vi "Counter - Count Edges.vi"() -> ()   [LabVIEW 2017]
doc: "本范例演示连续读回所有经计数器输入计算到的数字边沿的方法。\n\n关于将信号连接至DAQ设备的方法，可参考设备文档。"
uses:
  <vilib>/Utility/error.llb/DialogType.ctl
  <vilib>/DAQmx/read.llb/DAQmx Read (Counter U32 1Chan 1Samp).vi
  <vilib>/DAQmx/create/channels.llb/DAQmx Create Channel (CI-Count Edges).vi
  <vilib>/DAQmx/miscellaneous.llb/DAQmx Fill In Error Info.vi
  <resource>/objmgr/daqmx.rc
panel:
  in  "有效边沿":i32(ring)=10171 items=["上升"=10280, "下降"=10171]
  out "计数":u32
  in  "输入接线端":tag="PFI8"
  in  "计数器":tag="Dev1/ctr0"
  in  "触发类型":T1(tab)
  in  "边沿":i32(ring)=10280 items=["上升"=10280, "下降"=10171]
  in  "数字触发源":tag
  in  "暂停条件":i32(ring)=10192 items=["高"=10192, "低"=10214]
  in  "暂停触发源":tag
  in  "计数重置接线端":tag
  in  "边沿":i32(ring)=10280 items=["上升"=10280, "下降"=10171]
  in  "停止":bool
  in  "循环时间(ms)":u32=10
  # "采集数据"
  # "通道设置"
  # "定时\n设置"
  # "触发设置"
  # "如需配置并使用触发/计数重置，必须先在上面选择相应的选项卡。  有些硬件不支持上述选项－更多信息见设备的相应文档。"
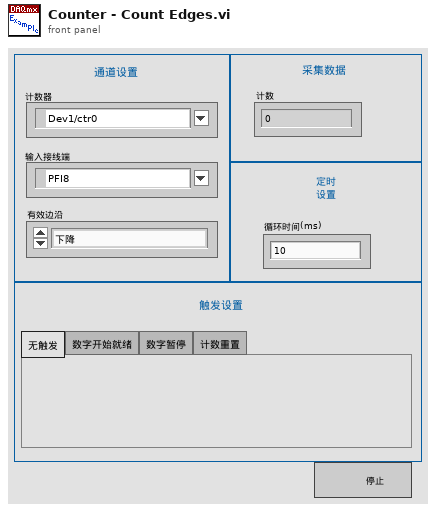
[diagram p1: front panel]
types:
  T1 = enum32{"No Trigger", "Digital Arm Start", "Digital Pause", "Count Reset"}
  T2 = typedef "DialogType.ctl" = u16
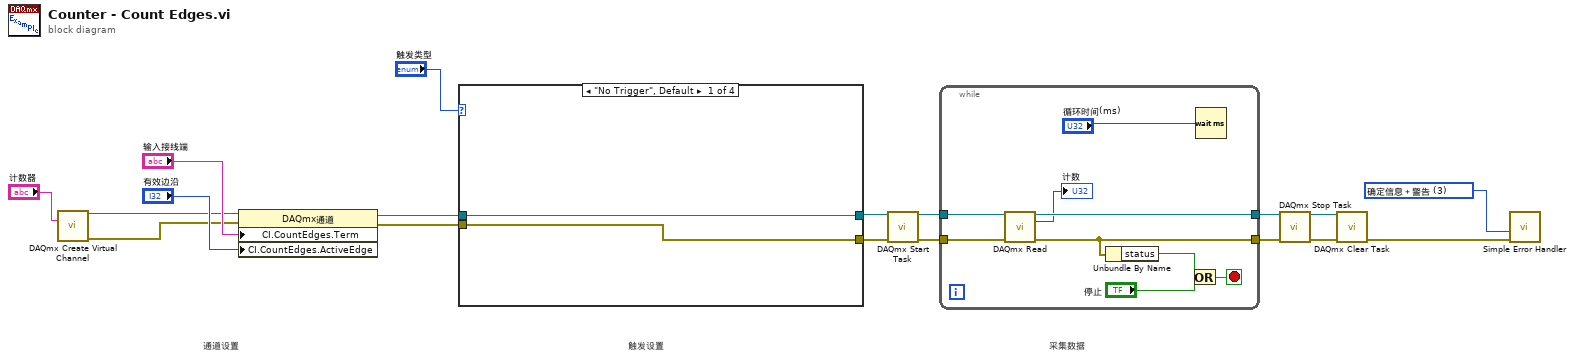
[diagram p0: block diagram]
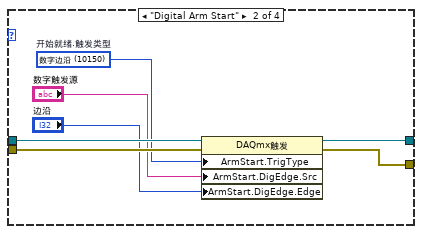
[diagram p2: hidden frame]
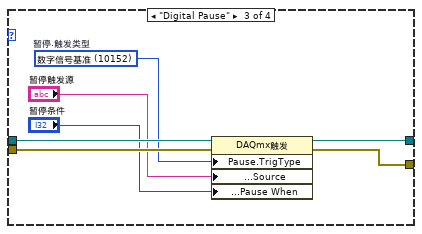
[diagram p3: hidden frame]
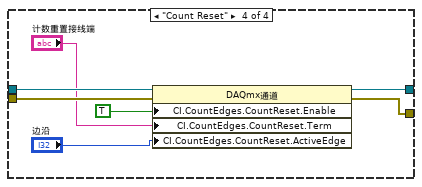
[diagram p4: hidden frame]
diagram:
  w1 = T2 3 items=["无对话框", "确定信息", "继续或停止信息", "确定信息＋警告", "继续/停止＋警告"] ("对话框类型（确定信息：1）")
  # "采集数据"
  # "触发设置"
  # "通道设置"
  n1 = call-poly <vilib>:"DAQmx Create Virtual Channel.vi"("counter"="计数器") -> ("task out"=w9:refnum<k21>, "error out"=w8:errorcluster)  [unwired: 13 in]
  n2 = property class="DAQmx通道"(reference=w9, error in=w8, "CI.CountEdges.Term"="输入接线端", "CI.CountEdges.ActiveEdge"="有效边沿") -> (reference out=w6:refnum<k21>, error out=w7:errorcluster)
  n3 = case shown="\"No Trigger\", Default" "触发类型" {
    tunnel: w6 -> [w20 w27 w34 w41]
    tunnel: w7 -> [w19 w24 w31 w38]
    tunnel: [w20 w26 w33 w40] -> w16
    tunnel: [w19 w25 w32 w39] -> w15
    frame "No Trigger", Default {
    }
    frame "Digital Arm Start" {
      w21 = 10150 items=["数字边沿"=10150, "无"=10230]  # 开始就绪.触发类型
      n4 = property class="DAQmx触发"(reference=w27, error in=w24, "ArmStart.TrigType"=w21, "ArmStart.DigEdge.Src"="数字触发源", "ArmStart.DigEdge.Edge"="边沿") -> (reference out=w26:refnum<k21>, error out=w25:errorcluster)
    }
    frame "Digital Pause" {
      w30 = 10152 items=["模拟信号基准"=10101, "模拟窗"=10103, "数字信号基准"=10152, "数字模式"=10398, "无"=10230]  # 暂停.触发类型
      n5 = property class="DAQmx触发"(reference=w34, error in=w31, "Pause.TrigType"=w30, "More:Pause:Digital Level:Source"="暂停触发源", "More:Pause:Digital Level:Pause When"="暂停条件") -> (reference out=w33:refnum<k21>, error out=w32:errorcluster)
    }
    frame "Count Reset" {
      n6 = property class="DAQmx通道"(reference=w41, error in=w38, "CI.CountEdges.CountReset.Enable"=TRUE ("计数器输入.边沿计数.计数重置.启用"), "CI.CountEdges.CountReset.Term"="计数重置接线端", "CI.CountEdges.CountReset.ActiveEdge"="边沿") -> (reference out=w40:refnum<k21>, error out=w39:errorcluster)
    }
  }
  n7 = call <vilib>:"DAQmx Start Task.vi"("task/channels in"=w16, "error in"=w15) -> ("task out"=w14:refnum<k21>, "error out"=w13:errorcluster)  [unwired: 12 in]
  n8 = while {
    tunnel: w14 -> [w50]
    tunnel: w13 -> [w49]
    tunnel: [w46] -> w4
    tunnel: [w47] -> w5
    stop <- w48 stop-if-true
    n9 = call-poly <vilib>:"DAQmx Read.vi"("task/channels in"=w50, "error in"=w49) -> ("task out"=w47:refnum<k21>, "data"=→"计数":u32, "error out"=w46:errorcluster)  [unwired: 11 in]
    n10 = Unbundle By Name(w46) -> ("status"=w45:bool)
    n11 = Or(x=w45, y="停止") -> (x .or. y?=w48:bool)
    n12 = Wait (ms)(milliseconds to wait="循环时间(ms)") -> ()  [unwired: 1 out]
  }
  n13 = call <vilib>:"DAQmx Stop Task.vi"("task/channels in"=w5, "error in"=w4) -> ("task out"=w2:refnum<k21>, "error out"=w3:errorcluster)  [unwired: 12 in]
  n14 = call <vilib>:"DAQmx Clear Task.vi"("task in"=w2, "error in"=w3) -> ("error out"=w12:errorcluster)  [unwired: 13 in]
  n15 = call <vilib>:"Simple Error Handler.vi"("type of dialog (OK msg:1)"=w1, "error in (no error)"=w12) -> ()  [unwired: 3 in, 5 out]
